vi "Open Webpage VIPM.vi"   [LabVIEW 2020]
uses:
  <vilib>/Platform/browser.llb/Open URL in Default Browser (string).vi
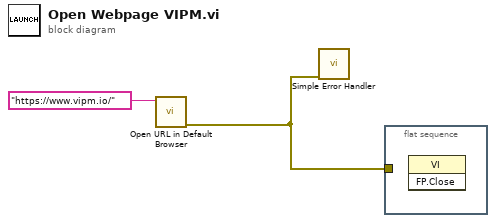
[diagram p0: block diagram]
diagram:
  n1 = call-poly <vilib>:"Open URL in Default Browser.vi"("URL"="https://www.vipm.io/") -> ("error out"=w1:errorcluster)  [unwired: 5 in, 1 out]
  n2 = call <vilib>:"Simple Error Handler.vi"("error in (no error)"=w1) -> ()  [unwired: 4 in, 5 out]
  n3 = flat-sequence {
    tunnel: w1 -> [_]
    frame #0 {
      n4 = invoke class="VI" method="FP.Close"() -> ()  [unwired: 3 in, 3 out]
    }
  }
